vi "Run Tests in UI.vi"(8 "error in (no error)":errorcluster, 10 "Path":path, 11 "Application":refnum<vi>) -> (0 "error out":errorcluster)   [LabVIEW 2020, in "Project Provider.lvlib"]
uses:
  Project Provider.lvlib
  Execution UI/User Interface.vi
  Execution UI/Execution UI.lvclass
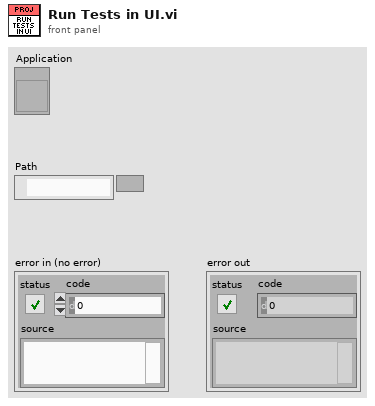
[diagram p1: front panel]
types:
  T1 = enum32{"Invalid", "Standard", "Closed", "Hidden", "Minimized", "Maximized"}
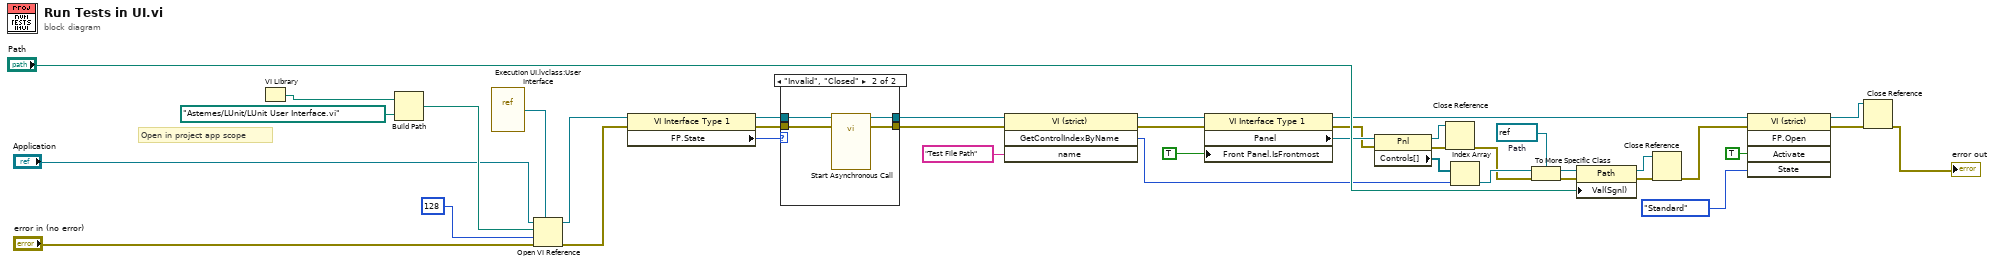
[diagram p0: block diagram]
diagram:
  w17 = refnum<vi> refnum  # Path
  # "Open in project app scope"
  n1 = VI Library() -> (path=w26:path)
  n2 = Build Path(base path=w26, name or relative path=path "Astemes/LUnit/LUnit User Interface.vi" ("Relative Path from 1 to 2")) -> (appended path=w34:path)
  n3 = vi-ref "Execution UI.lvclass:User Interface.vi"() -> (w25:refnum<vi>)
  n4 = Open VI Reference(type specifier VI Refnum (for type only)=w25, application reference (local)="Application", vi path=w34, options=128, error in (no error)="error in (no error)") -> (vi reference=w35:refnum<vi>, error out=w38:errorcluster)  [unwired: 1 in]
  n5 = property class="VI Interface Type 1"(reference=w35, error in=w38) -> (reference out=w27:refnum<vi>, error out=w28:errorcluster, "FP.State"=w5:T1)
  n6 = case shown="\"Invalid\", \"Closed\"" w5 {
    tunnel: w28 -> [w41 w45]
    tunnel: w27 -> [w40 w44]
    tunnel: [w41 w42] -> w4
    tunnel: [w40 w43] -> w3
    frame Default {
    }
    frame "Invalid", "Closed" {
      n7 = call-by-ref "Start Asynchronous Call"(reference=w44, error in=w45) -> (reference out=w43:refnum<vi>, error out=w42:errorcluster)  [unwired: 12 in]
    }
  }
  n8 = invoke class="VI (strict)" method="GetControlIndexByName"(reference=w3, error in=w4, "name"="Test File Path" ("Control Name")) -> (reference out=w21:refnum<vi>, error out=w11:errorcluster, "GetControlIndexByName"=w18:i32)  [unwired: 1 in, 1 out]
  n9 = property class="VI Interface Type 1"(reference=w21, error in=w11, "Front Panel.IsFrontmost"=TRUE ("Front Panel Window:Is Frontmost")) -> (reference out=w1:refnum<vi>, error out=w12:errorcluster, "Panel"=w22:refnum<vi>)
  n10 = property class="Pnl"(reference=w22, error in=w12) -> (reference out=w8:refnum<vi>, error out=w13:errorcluster, "Controls[]"=w19:refnum<vi>[])
  n11 = Close Reference(reference=w8, error in (no error)=w13) -> (error out=w9:errorcluster)
  n12 = Index Array(array=w19, index=w18) -> (element=w15:refnum<vi>)
  n13 = To More Specific Class(target class=w17, reference=w15, error in=w9) -> (specific class reference=w16:refnum<vi>, error out=w14:errorcluster)
  n14 = property class="Path"(reference=w16, error in=w14, "Val(Sgnl)"="Path") -> (reference out=w7:refnum<vi>, error out=w10:errorcluster)
  n15 = Close Reference(reference=w7, error in (no error)=w10) -> (error out=w2:errorcluster)
  n16 = invoke class="VI (strict)" method="FP.Open"(reference=w1, error in=w2, "Activate"=TRUE ("Activate?"), "State"=T1."Standard") -> (reference out=w33:refnum<vi>, error out=w31:errorcluster)  [unwired: 1 in, 3 out]
  n17 = Close Reference(reference=w33, error in (no error)=w31) -> (error out=→"error out":errorcluster)
